vi "Simulated Inactive DTCs.vi"() -> (3 "payload":u8[](array[numeric]))   [LabVIEW 2013, in "J1939.lvlib"]
uses:
  J1939.lvlib
  API Types/Convert DTCs Cluster.ctl
  <vilib>/xnet/xnet.llb/XNET Frame CAN.ctl
  <vilib>/xnet/xnet.llb/XNET Frame Type CAN.ctl
panel:
  out "Converted Value":T1={"Lamps"={"Malfunction Indicator"=0, "Red Stop"=1, "Amber Warning"=2, "Protect Lamp"=1}, "DTCs"=[{"SPN"=74273, "FMI"=3, "Occurrance"=36}, {"SPN"=75301, "FMI"=7, "Occurrance"=40}, {"SPN"=77865, "FMI"=17, "Occurrance"=50}], "Active?"=FALSE, "Address"=0, "timestamp"=timestamp(0 s since 1904-01-01)}
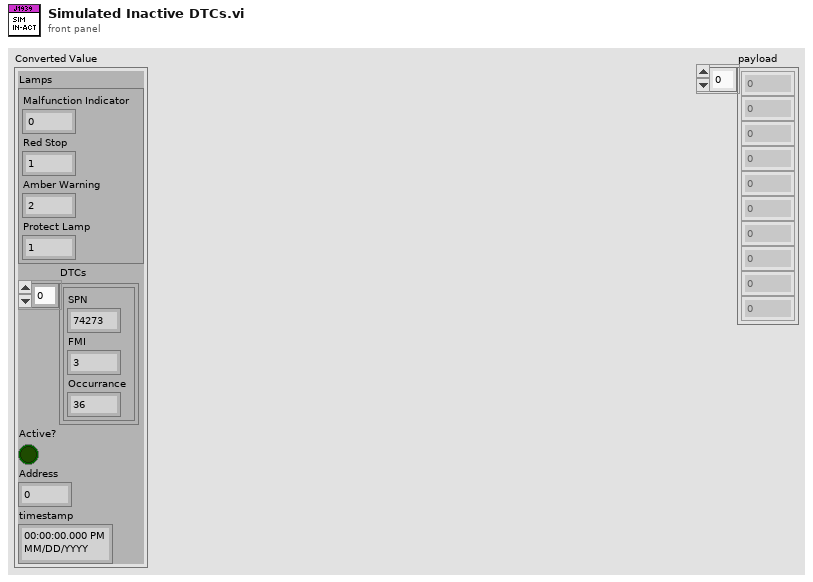
[diagram p1: front panel]
types:
  T1 = typedef "J1939.lvlib/Convert DTCs Cluster.ctl" = cluster{"Lamps":cluster{"Malfunction Indicator":u8, "Red Stop":u8, "Amber Warning":u8, "Protect Lamp":u8}, "DTCs":cluster{"SPN":u32, "FMI":u8, "Occurrance":u8}[], "Active?":bool, "Address":u8, "timestamp":timestamp}
  T2 = typedef "XNET Frame CAN.ctl" = cluster{"timestamp":timestamp, "payload":u8[], "identifier":u32, "type":T3, "extended?":bool, "echo?":bool}
  T3 = typedef "XNET Frame Type CAN.ctl" = u8
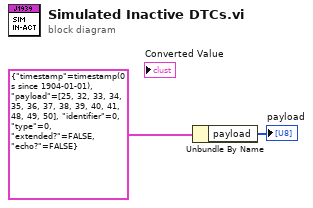
[diagram p0: block diagram]
diagram:
  n1 = Unbundle By Name(T2 {"timestamp"=timestamp(0 s since 1904-01-01), "payload"=[25, 32, 33, 34, 35, 36, 37, 38, 39, 40, 41, 48, 49, 50], "identifier"=0, "type"=0, "extended?"=FALSE, "echo?"=FALSE} ("value")) -> ("payload"=→"payload":u8[])
